vi "TSM SSC Digital Stream HRAM Results.vi"(0 "Digital TSM In":T3, 11 "error in":errorcluster) -> (4 "Digital TSM Out":T3, 6 "Per-Site Cycle Information":T1[][](array[typedef]) {"actual pin states" items=["0"=0, "1"=1, "L"=3, "H"=4, "X"=5, "M"=6, "V"=7, "D"=8, "E"=9, "Not A Pin State"=254, "Pin State Not Acquired"=255]; "expected pin states" items=["0"=0, "1"=1, "L"=3, "H"=4, "X"=5, "M"=6, "V"=7, "D"=8, "E"=9, "Not A Pin State"=254, "Pin State Not Acquired"=255]}, 8 "Per-Site Scan Cycle Numbers":i64[][](array[numeric]) format="%.0x", 15 "error out":errorcluster)   [LabVIEW 2020]
doc: "Fetches a defined number of samples for the sites connected to the specified pin(s) and pin group(s). This VI only returns data from sites that are enabled when fetch is called. Returns an array of per-site per-sample data where rows correspond to sites and columns correspond to samples."
uses:
  TSM/TSM SSC Digital.ctl
  <vilib>/NI_TestStand_SemiconductorModule/NI_TestStand_Semiconductor_Module.lvlibp/PinMap/Digital Pattern/PinQueryContext/DigitalPatternPinQueryContext.lvclass
  SSC Digital/SSC Digital.ctl
  <instrlib>/niDigital/niDigital.llb/niDigital History RAM Cycle Information (1D Pin States).ctl
  <instrlib>/niDigital/niDigital.llb/niDigital Pin State.ctl
  Shared SubVIs/Site List to Site Numbers.vi
  Shared SubVIs/Trim Whitespace [Inlined].vi
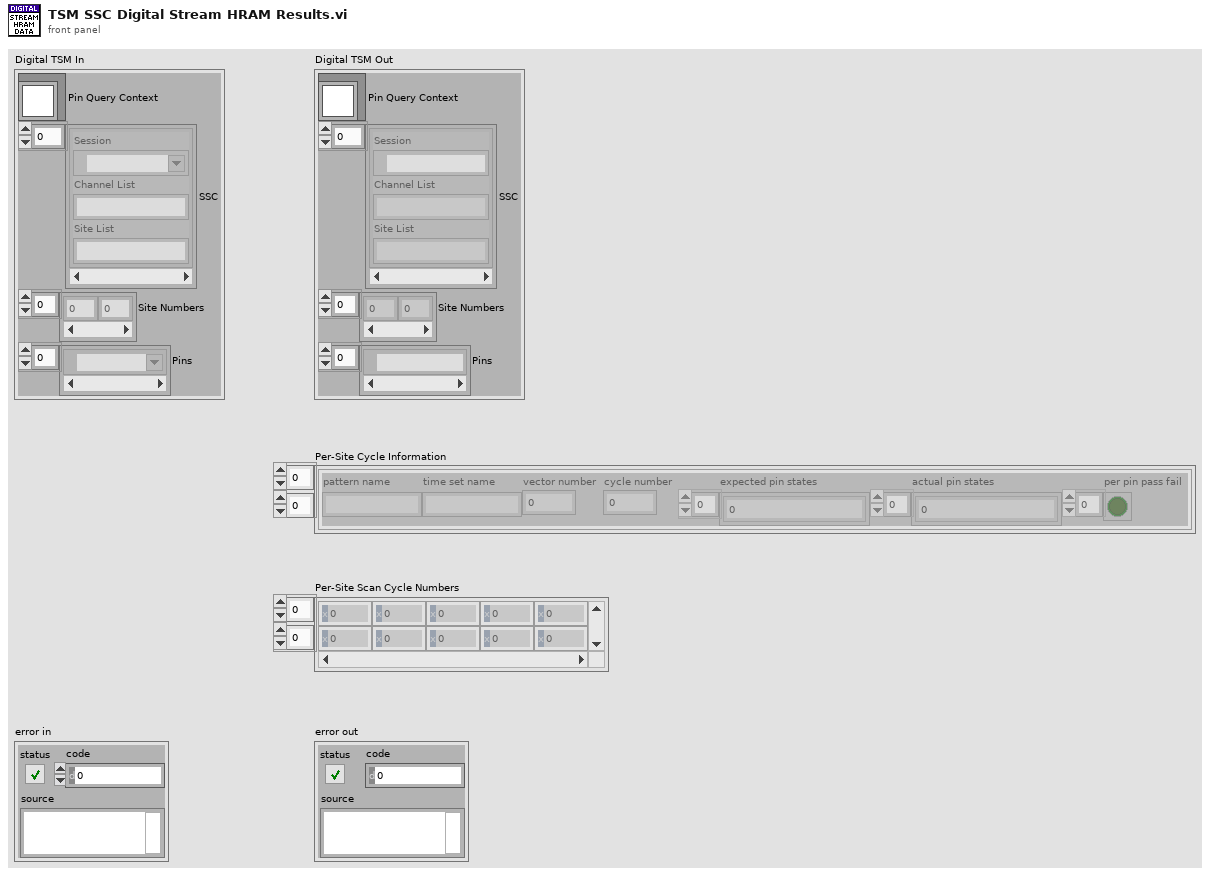
[diagram p1: front panel]
types:
  T1 = typedef "niDigital History RAM Cycle Information (1D Pin States).ctl" = cluster{"pattern name":string, "time set name":string, "vector number":i64, "cycle number":i64, "expected pin states":T2[], "actual pin states":T2[], "per pin pass fail":bool[]}
  T2 = typedef "niDigital Pin State.ctl" = u8
  T3 = typedef "TSM SSC Digital.ctl" = cluster{"Pin Query Context":refnum<class "DigitalPatternPinQueryContext.lvclass">, "SSC":T4[], "Site Numbers":i32[], "Pins":tag[]}
  T4 = typedef "SSC Digital.ctl" = cluster{"Session":refnum<k15>, "Channel List":string, "Site List":string}
  T5 = typedef "Digital 1D Location Array in a Cluster.ctl" = cluster{"Digital 1D Location Array":i32[]}
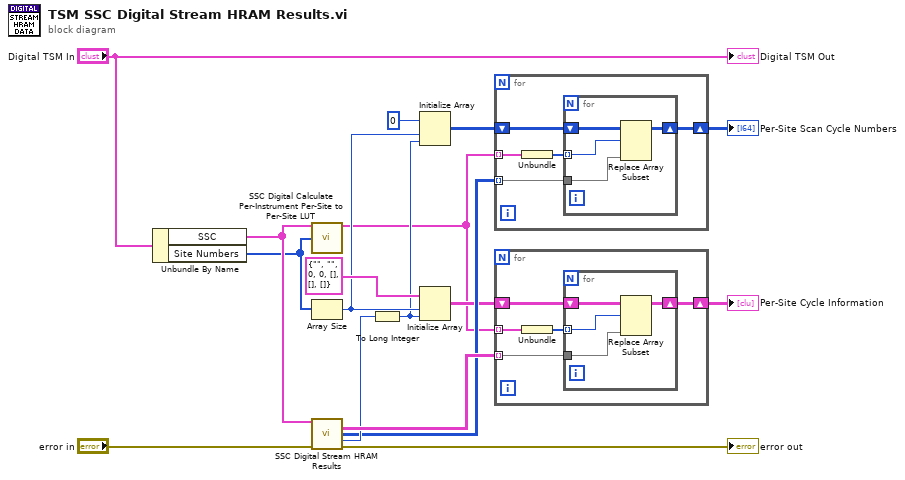
[diagram p0: block diagram]
diagram:
  n1 = Unbundle By Name("Digital TSM In") -> ("SSC"=w15:T4[], "Site Numbers"=w13:i32[])
  n2 = call "SSC Digital Calculate Per-Instrument Per-Site to Per-Site LUT.vi"("Digital SSC In"=w15, "Sites"=w13) -> ("Per-Instrument Per-Site to Per-Site LUT"=w1:T5[])  [unwired: 13 in]
  n3 = Array Size(array=w13) -> (size(s)=w6:i32)
  n4 = call "SSC Digital Stream HRAM Results.vi"("Digital SSC in"=w15, "error in"="error in") -> ("per-instrument per-site cycle information"=w8:T1[][], "per-instrument per-site scan cycle numbers"=w3:i64[][], "number of samples"=w7:i64, "error out"=→"error out":errorcluster)  [unwired: 9 in, 1 out]
  n5 = To Long Integer(number=w7) -> (32bit integer=w5:i32)
  n6 = Initialize Array(i64 0, w6, w5) -> (w4:i64[][])
  n7 = Initialize Array(T1 {"pattern name"="", "time set name"="", "vector number"=0, "cycle number"=0, "expected pin states"=[], "actual pin states"=[], "per pin pass fail"=[]} ("cycle information (1D Pin States)"), w6, w5) -> (w2:T1[][])
  n8 = for {
    shift-right: [w21] -> w10
    shift-left: w4 -> [w22]
    tunnel: w3 -> [w20] mode=indexing
    tunnel: w1 -> [w19] mode=indexing
    n9 = Unbundle(w19) -> ("Digital 1D Location Array"=w18:i32[])
    n10 = for {
      shift-right: [w25] -> w21
      shift-left: w22 -> [w26]
      tunnel: w20 -> [w24]
      tunnel: w18 -> [w23] mode=indexing
      n11 = Replace Array Subset(array=w26, new element=w24, index (row)=w23) -> (w25:i64[][])  [unwired: 1 in]
    }
  }
  "Per-Site Scan Cycle Numbers" <- w10
  n12 = for {
    shift-right: [w30] -> w9
    shift-left: w2 -> [w31]
    tunnel: w8 -> [w29] mode=indexing
    tunnel: w1 -> [w28] mode=indexing
    n13 = Unbundle(w28) -> ("Digital 1D Location Array"=w27:i32[])
    n14 = for {
      shift-right: [w34] -> w30
      shift-left: w31 -> [w35]
      tunnel: w29 -> [w33]
      tunnel: w27 -> [w32] mode=indexing
      n15 = Replace Array Subset(array=w35, new element=w33, index (row)=w32) -> (w34:T1[][])  [unwired: 1 in]
    }
  }
  "Per-Site Cycle Information" <- w9
  "Digital TSM Out" <- "Digital TSM In"
